vi "PFD_main.vi"(11 "Refresh Rate (Hz)":u32=60) -> ()   [LabVIEW 2023]
panel:
  out "x/y":dbl
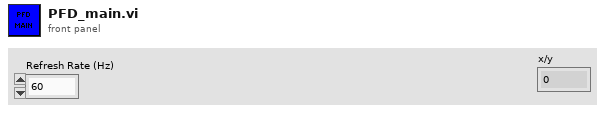
[diagram p1: front panel]
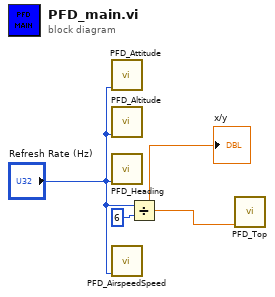
[diagram p0: block diagram]
diagram:
  n1 = call "PFD_Attitude.vi"("Refresh Rate (Hz)"="Refresh Rate (Hz)") -> ()  [unwired: 9 in, 2 out]
  n2 = call "PFD_Altitude.vi"("Refresh Rate (Hz)"="Refresh Rate (Hz)") -> ()  [unwired: 8 in, 3 out]
  n3 = call "PFD_Heading.vi"("Refresh Rate (Hz)"="Refresh Rate (Hz)") -> ()  [unwired: 7 in, 4 out]
  n4 = call "PFD_AirspeedSpeed.vi"("Refresh Rate (Hz)"="Refresh Rate (Hz)") -> ()  [unwired: 9 in, 2 out]
  n5 = Divide(x="Refresh Rate (Hz)", y=u32 6) -> (x/y=w1:dbl)
  "x/y" <- w1
  n6 = call "PFD_Top.vi"("Refresh Rate (Hz)"=w1) -> ()  [unwired: 9 in, 2 out]
